vi "StopSignal-AsNotifier.vi"(8 "error in (no error)":errorcluster, 11 "StopSignal":T1) -> (0 "error out":errorcluster, 3 "StopNotifier":refnum<notifier>)   [LabVIEW 2017, in "StopSignal.lvlib"]
uses:
  StopSignal.lvlib
  Typedef/StopSignal.ctl
  Typedef/def-StopReason.ctl
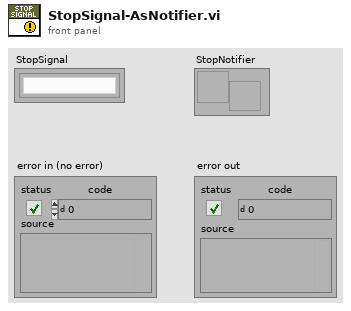
[diagram p1: front panel]
types:
  T1 = typedef "StopSignal.lvlib/StopSignal.ctl" = refnum<k1>
  T2 = typedef "StopSignal.lvlib/Def-StopSignalData.ctl" = cluster{"StopEvent":refnum<user-event>, "StopNotifier":refnum<notifier>, "StopReason":T3}
  T3 = typedef "StopSignal.lvlib/def-StopReason.ctl" = cluster{"Reason":string, "timestamp":timestamp}
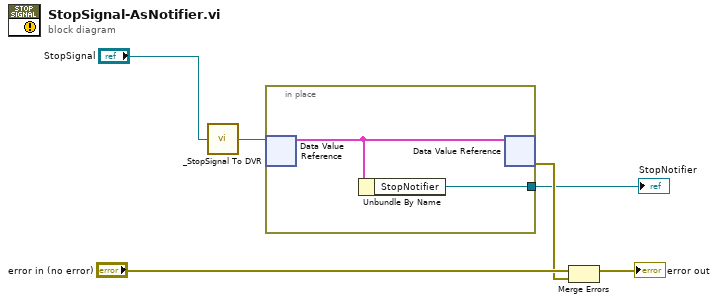
[diagram p0: block diagram]
diagram:
  n1 = call "_StopSignal To DVR.vi"("Refnum in"="StopSignal") -> ("Data Value Reference out"=w4:refnum<data-value>)
  n2 = in-place {
    in-place-border: [w7] -> w1
    n3 = in-place-dvr #1(w4) -> (w8:T2)  [unwired: 1 out]
    n4 = Unbundle By Name(w8) -> ("StopNotifier"=w7:refnum<notifier>)
    n5 = in-place-dvr #1(w8) -> (w2:errorcluster)  [unwired: 1 out]
  }
  "StopNotifier" <- w1
  n6 = Merge Errors("error in (no error)", w2) -> (→"error out":errorcluster)
